vi "Read Display Order.vi"(8 "error in (no error)":errorcluster, 11 "Item in":refnum<class "Item.lvclass">) -> (0 "error out":errorcluster, 2 "Display Order":i32, 3 "Item out":refnum<class "Item.lvclass">)   [LabVIEW 2020, in "VI Properties Editor.lvlib" / "Item.lvclass"]
doc: "Gets or sets the display order of the item, as it appears in the top-level project, library, or class it was loaded from."
uses:
  Item.lvclass
  Item.lvclass/Item.ctl
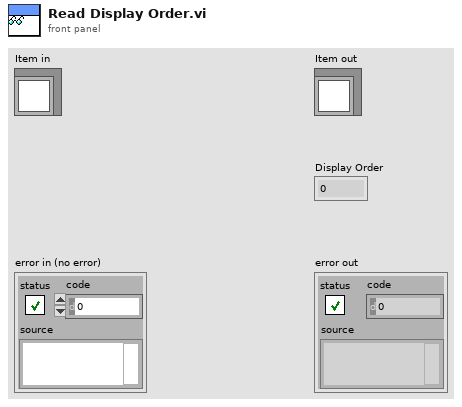
[diagram p1: front panel]
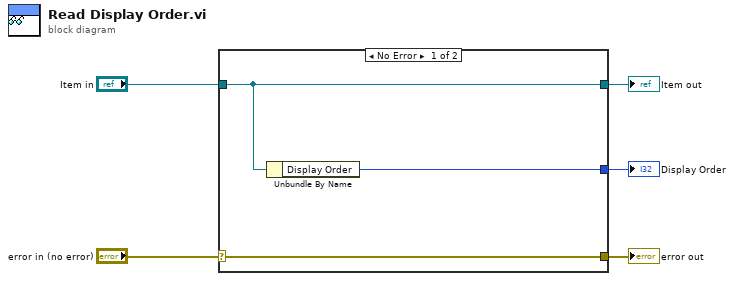
[diagram p0: block diagram]
diagram:
  n1 = case shown="No Error" "error in (no error)" {
    selector: "error in (no error)" -> [w8 w9]
    tunnel: [w8 w9] -> w4
    tunnel: [w7 w10] -> w2
    tunnel: "Item in" -> [w7 w10]
    tunnel: [w6 _] -> w1
    frame No Error {
      n2 = Unbundle By Name(w7) -> ("Display Order"=w6:i32)
    }
    frame Error {
    }
  }
  "error out" <- w4
  "Item out" <- w2
  "Display Order" <- w1
